vi "Reorder Display Elements By Layer.vi"(8 "Error In":errorcluster, 11 "Display In":refnum<class "Display.lvclass">) -> (0 "Error Out":errorcluster, 3 "Display Out":refnum<class "Display.lvclass">)   [LabVIEW 2019, in "Display.lvclass"]
uses:
  Display.lvclass
  Display Element/Display Element.lvclass
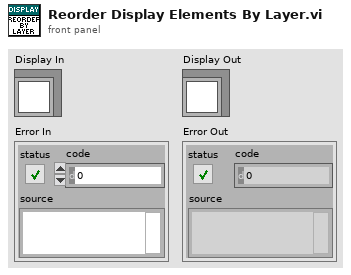
[diagram p1: front panel]
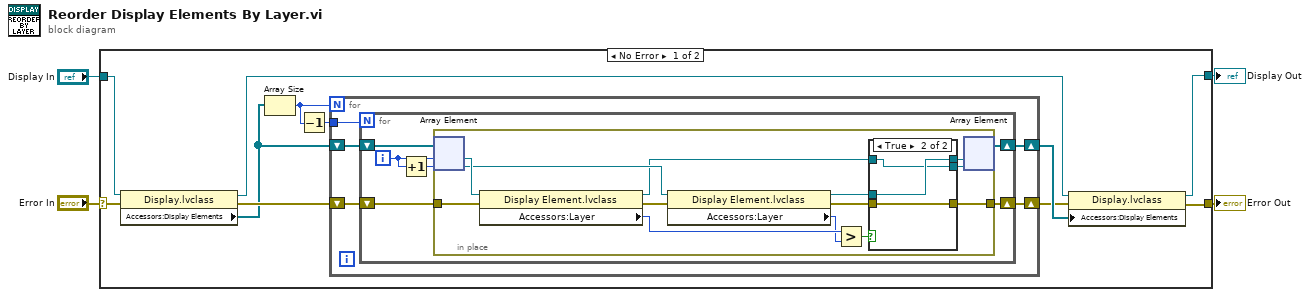
[diagram p0: block diagram]
diagram:
  n1 = case shown="No Error" "Error In" {
    selector: "Error In" -> [w14 w46]
    tunnel: "Display In" -> [w15 w47]
    tunnel: [w8 w47] -> w2
    tunnel: [w9 w46] -> w1
    frame No Error {
      n2 = property class="Display.lvclass"(reference=w15, error in=w14) -> (reference out=w12:refnum<class "Display.lvclass">, error out=w13:errorcluster, "Accessors:Display Elements"=w7:refnum<class "Display Element.lvclass">[])
      n3 = Array Size(array=w7) -> (size(s)=w6:i32)
      n4 = Decrement(x=w6) -> (x-1=w5:i32)
      n5 = for {
        N: w6 -> [_]
        shift-right: [w17] -> w10
        shift-left: w13 -> [w19]
        shift-right: [w18] -> w11
        shift-left: w7 -> [w20]
        tunnel: w5 -> [w16]
        n6 = for {
          N: w16 -> [_]
          shift-right: [w21] -> w17
          shift-left: w19 -> [w22]
          shift-right: [w25] -> w18
          shift-left: w20 -> [w26]
          i -> [w24]
          n7 = Increment(x=w24) -> (x+1=w23:i32)
          n8 = in-place {
            in-place-border: w22 -> [w38]
            in-place-border: [w27] -> w21
            n9 = in-place-array #1(w26, w24, w23) -> (w39:refnum<class "Display Element.lvclass">, w37:refnum<class "Display Element.lvclass">)
            n10 = property class="Display Element.lvclass"(reference=w39, error in=w38) -> (reference out=w32:refnum<class "Display Element.lvclass">, error out=w36:errorcluster, "Accessors:Layer"=w35:u32)
            n11 = property class="Display Element.lvclass"(reference=w37, error in=w36) -> (reference out=w31:refnum<class "Display Element.lvclass">, error out=w28:errorcluster, "Accessors:Layer"=w34:u32)
            n12 = Greater?(x=w35, y=w34) -> (0:w33:bool)
            n13 = case shown="True" w33 {
              tunnel: w32 -> [w42 w44]
              tunnel: w31 -> [w41 w45]
              tunnel: [w42 w45] -> w30
              tunnel: [w41 w44] -> w29
              tunnel: w28 -> [w40 w43]
              tunnel: [w40 w43] -> w27
              frame False {
              }
              frame True {
              }
            }
            n14 = in-place-array #1(w30, w29) -> (w25:refnum<class "Display Element.lvclass">[])  [unwired: 2 out]
          }
        }
      }
      n15 = property class="Display.lvclass"(reference=w12, error in=w10, "Accessors:Display Elements"=w11) -> (reference out=w8:refnum<class "Display.lvclass">, error out=w9:errorcluster)
    }
    frame Error {
    }
  }
  "Display Out" <- w2
  "Error Out" <- w1
